vi "EGSE Comms.vi"() -> ()   [LabVIEW 2020]
uses:
  Type Definitions/Data Frame.ctl
  Type Definitions/Data Frame Header.ctl
  Type Definitions/Payload Class.ctl
  Type Definitions/Device Parameters.ctl
  Type Definitions/Device.ctl
  <vilib>/dex/Stream Element Allocation Mode.ctl
panel:
  out "data out":T1 {"CRC" format="%08x"; "Frame Header"."Options" format="%016b"; "Frame Header"."Time" format="%^<%I:%M:%S%3u %p\n%m/%d/%Y %Z>T"; "Frame Header"."Sync" format="%08x"}
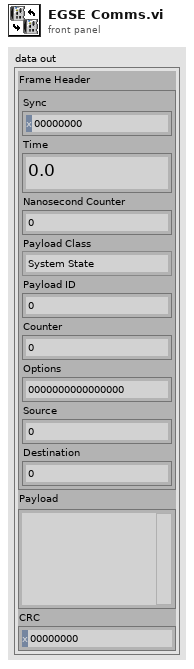
[diagram p1: front panel]
types:
  T1 = typedef "Data Frame.ctl" = cluster{"Frame Header":T2, "Payload":string, "CRC":u32}
  T2 = typedef "Data Frame Header.ctl" = cluster{"Sync":u32, "Time":dbl, "Nanosecond Counter":i64, "Payload Class":T3, "Payload ID":u16, "Counter":u32, "Options":u32, "Source":i32, "Destination":i32}
  T3 = typedef "Payload Class.ctl" = enum16{"System State", "Parameters", "Metadata", "Software Monitor", "Data", "Commands"}
  T4 = typedef "Device Parameters.ctl" = cluster{"Device":T5}
  T5 = typedef "Device.ctl" = enum32{"None", "Exec", "Aux1", "Aux2", "Aux3"}
  T6 = typedef "Stream Element Allocation Mode.ctl" = u32
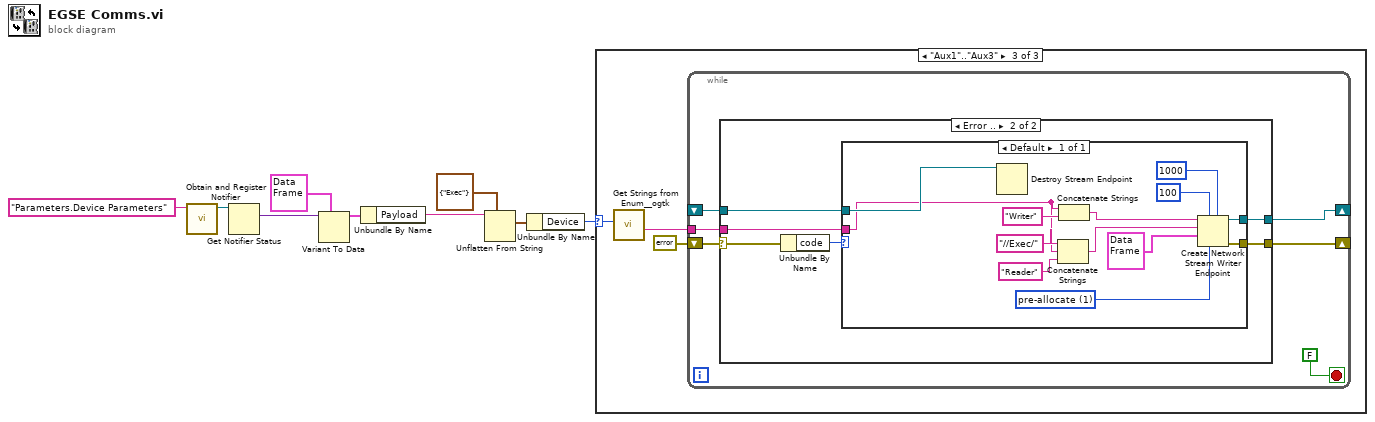
[diagram p0: block diagram]
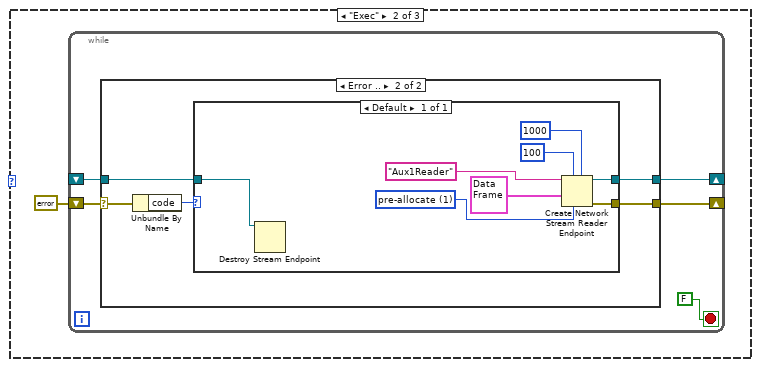
[diagram p3: hidden frame]
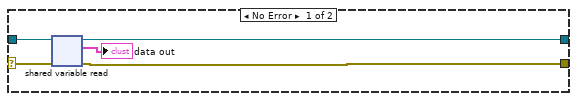
[diagram p4: hidden frame]
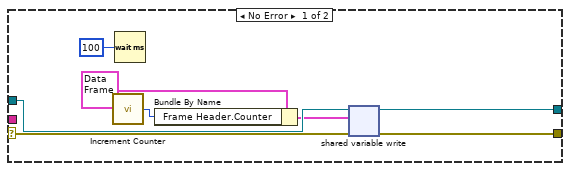
[diagram p5: hidden frame]
diagram:
  n1 = call "Obtain and Register Notifier.vi"("name (unnamed)"="Parameters.Device Parameters") -> ("notifier out"=w8:refnum<notifier>)  [unwired: 8 in, 2 out]
  n2 = Get Notifier Status(notifier=w8) -> (current notification=w7:variant)  [unwired: 1 in, 4 out]
  n3 = Variant To Data(type=T1 {"Frame Header"={"Sync"=0, "Time"=0.0, "Nanosecond Counter"=0, "Payload Class"=enum."System State", "Payload ID"=0, "Counter"=0, "Options"=0, "Source"=0, "Destination"=0}, "Payload"="", "CRC"=0} ("Frame"), Variant=w7) -> (data=w5:T1)  [unwired: 1 in, 1 out]
  n4 = Unbundle By Name(w5) -> ("Payload"=w4:string)
  n5 = Unflatten From String(type=T4 {"Device"=enum."Exec"} ("Device Parameters"), binary string=w4) -> (value=w2:T4)  [unwired: 3 in, 2 out]
  n6 = Unbundle By Name(w2) -> ("Device"=w1:T5)
  n7 = case shown="\"Aux1\"..\"Aux3\"" w1 {
    selector: w1 -> [_ _ w35]
    frame "None", Default {
    }
    frame "Exec" {
      n8 = while {
        shift-right: [w15] -> _
        shift-left: errorcluster {"status"=TRUE, "code"=0, "source"=""} ("error out") -> [w14]
        shift-right: [w13] -> _
        shift-left: _ -> [w12]
        stop <- FALSE stop-if-true
        n9 = case shown="Error .." w14 {
          selector: w14 -> [w17 w23]
          tunnel: [w18 w25] -> w15
          tunnel: [w19 w24] -> w13
          tunnel: w12 -> [w20 w21]
          frame No Error {
            n10 = shared-variable-read(w20, w17) -> (w19:refnum<k21>, w18:errorcluster, →"data out":T1)  [unwired: 1 in, 1 out]
          }
          frame Error {
            n11 = Unbundle By Name(w23) -> ("code"=w22:i32)
            n12 = case shown="Default" w22 {
              tunnel: [w33] -> w25
              tunnel: [w27] -> w24
              tunnel: w21 -> [w26]
              frame Default {
                w29 = T6 1 items=["allocate as needed", "pre-allocate"] ("element allocation mode")
                n13 = Destroy Stream Endpoint(11:w26) -> ()  [unwired: 1 in, 1 out]
                n14 = Create Network Stream Reader Endpoint(5:1000 ("timeout in ms (-1)"), 6:w29, 7:100 ("reader buffer size"), 9:T1 {"Frame Header"={"Sync"=0, "Time"=0.0, "Nanosecond Counter"=0, "Payload Class"=enum."System State", "Payload ID"=0, "Counter"=0, "Options"=0, "Source"=0, "Destination"=0}, "Payload"="", "CRC"=0} ("Frame"), 11:"Aux1Reader" ("reader name")) -> (0:w33:errorcluster, 3:w27:refnum<k21>)  [unwired: 2 in]
              }
            }
          }
        }
      }
    }
    frame "Aux1".."Aux3" {
      n15 = call <userlib>:"Get Strings from Enum__ogtk.vi"("Enum"=w35) -> ("String Value"=w34:string)  [unwired: 7 in, 3 out]
      n16 = while {
        shift-right: [w42] -> _
        shift-left: errorcluster {"status"=TRUE, "code"=0, "source"=""} ("error out") -> [w41]
        shift-right: [w40] -> _
        shift-left: _ -> [w39]
        tunnel: w34 -> [w37]
        stop <- FALSE stop-if-true
        n17 = case shown="Error .." w41 {
          selector: w41 -> [w47 w54]
          tunnel: [w46 w56] -> w42
          tunnel: [w48 w55] -> w40
          tunnel: w39 -> [w49 w52]
          tunnel: w37 -> [_ w51]
          frame No Error {
            n18 = call "Increment Counter.vi"() -> ("Count"=w45:i32)  [unwired: 5 in]
            n19 = Wait (ms)(milliseconds to wait=u32 100) -> ()  [unwired: 1 out]
            n20 = Bundle By Name(cluster=T1 {"Frame Header"={"Sync"=0, "Time"=0.0, "Nanosecond Counter"=0, "Payload Class"=enum."System State", "Payload ID"=0, "Counter"=0, "Options"=0, "Source"=0, "Destination"=0}, "Payload"="", "CRC"=0} ("Frame"), "Frame Header.Counter"=w45) -> (w44:T1)
            n21 = shared-variable-write(w49, w47, w44) -> (w48:refnum<k21>, w46:errorcluster)  [unwired: 1 in, 1 out]
          }
          frame Error {
            n22 = Unbundle By Name(w54) -> ("code"=w53:i32)
            n23 = case shown="Default" w53 {
              tunnel: [w64] -> w56
              tunnel: [w65] -> w55
              tunnel: w52 -> [w63]
              tunnel: w51 -> [w59]
              frame Default {
                w68 = T6 1 items=["allocate as needed", "pre-allocate"] ("element allocation mode")
                n24 = Destroy Stream Endpoint(11:w63) -> ()  [unwired: 1 in, 1 out]
                n25 = Concatenate Strings("//Exec/" ("string"), w59, "Reader" ("string")) -> (w57:string)
                n26 = Concatenate Strings(w59, "Writer" ("string")) -> (w61:string)
                n27 = Create Network Stream Writer Endpoint(5:1000 ("timeout in ms (-1)"), 6:w68, 7:100 ("reader buffer size"), 9:T1 {"Frame Header"={"Sync"=0, "Time"=0.0, "Nanosecond Counter"=0, "Payload Class"=enum."System State", "Payload ID"=0, "Counter"=0, "Options"=0, "Source"=0, "Destination"=0}, "Payload"="", "CRC"=0} ("Frame"), 10:w57, 11:w61) -> (0:w64:errorcluster, 3:w65:refnum<k21>)  [unwired: 1 in]
              }
            }
          }
        }
      }
    }
  }
